vi "Get Block Images (SubVI).vi"(10 "Full Image In":u8[][](array[numeric]), 11 "Current Table":i32[][](array[numeric])) -> (2 "Block Annotation Location":i32[][](array[numeric]), 3 "Block Image":u8[][](array[numeric]))   [LabVIEW 2015]
uses:
  <vilib>/vision/NI_Vision_Development_Module.lvlib
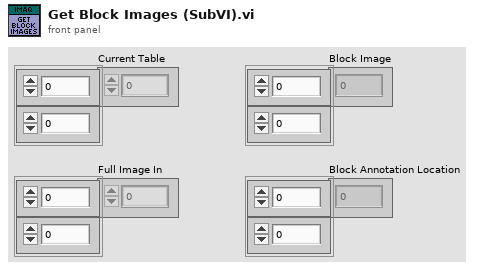
[diagram p1: front panel]
types:
  T1 = typedef "IMAQ Image.ctl" = refnum<image>
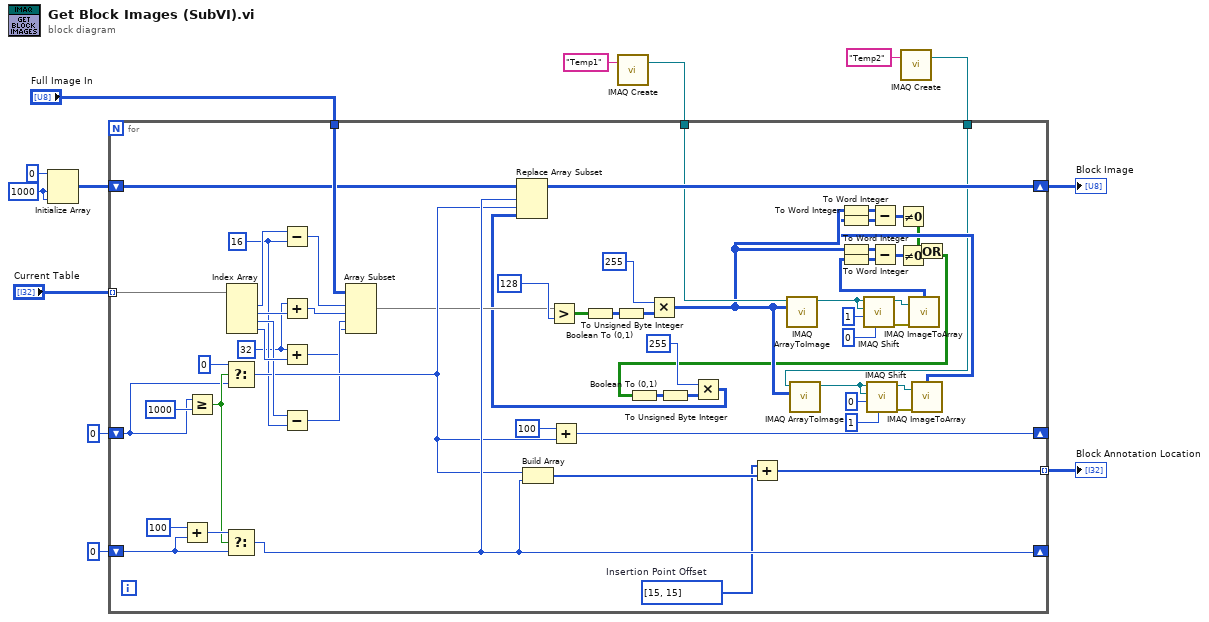
[diagram p0: block diagram]
diagram:
  w6 = 1000 ("dimension size")
  n1 = Initialize Array(u8 0 ("element"), w6, w6) -> (w5:u8[][])
  n2 = call "IMAQ Create"("Image Name"="Temp1") -> ("New Image"=w3:T1)  [unwired: 4 in, 1 out]
  n3 = call "IMAQ Create"("Image Name"="Temp2") -> ("New Image"=w2:T1)  [unwired: 4 in, 1 out]
  n4 = for {
    tunnel: "Current Table" -> [w44] mode=indexing
    tunnel: "Full Image In" -> [w75]
    shift-right: [w45] -> w9
    shift-left: w5 -> [w66]
    shift-right: [w63] -> _
    shift-left: 0 -> [w61]
    shift-right: [w59] -> _
    shift-left: 0 -> [w60]
    tunnel: [w57] -> w12 mode=indexing
    tunnel: w3 -> [w41]
    tunnel: w2 -> [w14]
    w50 = 32 ("x")
    w53 = 16 ("x")
    w56 = i32[] [15, 15]  # Insertion Point Offset
    n5 = Add(x=100, y=w60) -> (x+y=w68:i32)
    n6 = Greater Or Equal?(x=w61, y=1000) -> (x >= y?=w67:bool)
    n7 = Select(t=0, s=w67, f=w61) -> (s? t:f=w58:i32)
    n8 = Select(t=w68, s=w67, f=w60) -> (s? t:f=w59:i32)
    n9 = Index Array(array=w44) -> (element #1=w64:i32, element #2=w73:i32, element #3=w65:i32, element #4=w74:i32)  [unwired: 4 in]
    n10 = Subtract(x=w64, y=w53) -> (x-y=w55:i32)
    n11 = Add(x=w50, y=w73) -> (x+y=w52:i32)
    n12 = Add(x=w50, y=w74) -> (x+y=w51:i32)
    n13 = Subtract(x=w65, y=w53) -> (x-y=w54:i32)
    n14 = Array Subset(array=w75, index (row)=w55, length (row)=w52, index (col)=w54, length (col)=w51) -> (w46:u8[][])
    n15 = Build Array(w58, w59) -> (w62:i32[])
    n16 = Greater?(x=w46, y=u8 128 ("x")) -> (0:w49:bool[][])
    n17 = Add(x=100, y=w58) -> (x+y=w63:i32)
    n18 = Boolean To (0,1)(Boolean=w49) -> (0, 1=w47:i16[][])
    n19 = To Unsigned Byte Integer(number=w47) -> (unsigned 8bit integer=w43:u8[][])
    n20 = Multiply(x=u8 255, y=w43) -> (x*y=w18:u8[][])
    n21 = Add(x=w56, y=w62) -> (x+y=w57:i32[])
    n22 = call "IMAQ ArrayToImage"("Image Pixels (U8)"=w18, "Image"=w41) -> ("Image Out"=w40:T1)  [unwired: 8 in, 1 out]
    n23 = call "IMAQ ArrayToImage"("Image Pixels (U8)"=w18, "Image"=w14) -> ("Image Out"=w22:T1)  [unwired: 8 in, 1 out]
    n24 = To Word Integer(number=w18) -> (16bit integer=w19:i16[][])
    n25 = To Word Integer(number=w18) -> (16bit integer=w37:i16[][])
    n26 = call "IMAQ Shift"("YOffset"=0, "XOffset"=1, "Image Dst"=w40, "Image Src"=w40) -> ("error out"=w38:errorcluster, "Image Dst Out"=w29:T1)  [unwired: 6 in]
    n27 = call "IMAQ Shift"("YOffset"=1, "XOffset"=0, "Image Dst"=w22, "Image Src"=w22) -> ("error out"=w24:errorcluster, "Image Dst Out"=w25:T1)  [unwired: 6 in]
    n28 = call "IMAQ ImageToArray"("error in (no error)"=w38, "Image"=w29) -> ("Image Pixels (U8)"=w28:u8[][])  [unwired: 2 in, 4 out]
    n29 = To Word Integer(number=w28) -> (16bit integer=w36:i16[][])
    n30 = Subtract(x=w37, y=w36) -> (x-y=w35:i16[][])
    n31 = Not Equal To 0?(x=w35) -> (x != 0?=w31:bool[][])
    n32 = call "IMAQ ImageToArray"("error in (no error)"=w24, "Image"=w25) -> ("Image Pixels (U8)"=w17:u8[][])  [unwired: 2 in, 4 out]
    n33 = To Word Integer(number=w17) -> (16bit integer=w20:i16[][])
    n34 = Subtract(x=w19, y=w20) -> (x-y=w21:i16[][])
    n35 = Not Equal To 0?(x=w21) -> (x != 0?=w15:bool[][])
    n36 = Or(x=w15, y=w31) -> (x .or. y?=w16:bool[][])
    n37 = Boolean To (0,1)(Boolean=w16) -> (0, 1=w32:i16[][])
    n38 = To Unsigned Byte Integer(number=w32) -> (unsigned 8bit integer=w33:u8[][])
    n39 = Multiply(x=u8 255, y=w33) -> (x*y=w30:u8[][])
    n40 = Replace Array Subset(array=w66, new element=w30, index (row)=w59, index (col)=w58) -> (w45:u8[][])
  }
  "Block Annotation Location" <- w12
  "Block Image" <- w9
